vi "XNETsignal2String.vi"(0 "DBC_XnetSignal":refnum<k21>) -> (14 "X-netString":string)   [LabVIEW 2020]
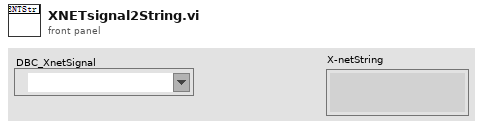
[diagram p1: front panel]
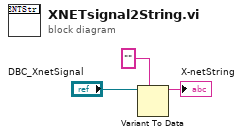
[diagram p0: block diagram]
diagram:
  n1 = Variant To Data(type="", Variant="DBC_XnetSignal") -> (data=→"X-netString":string)  [unwired: 1 in, 1 out]
